vi "get_linearised.vi"(8 "error in (no error)":errorcluster, 11 "ImageCollection in":refnum<class "ImageCollection.lvclass">) -> (0 "error out":errorcluster, 2 "pixels":dbl[](array[numeric]), 3 "ImageCollection out":refnum<class "ImageCollection.lvclass">)   [LabVIEW 2010, in "ImageCollection.lvclass"]
uses:
  ImageCollection.lvclass
  Image/Image/Image.lvclass
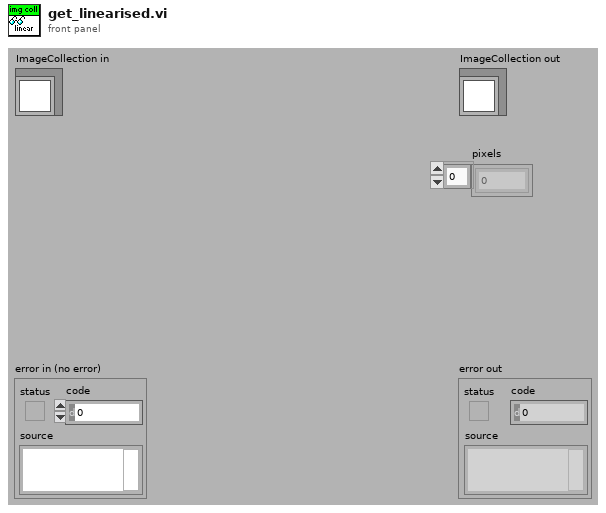
[diagram p1: front panel]
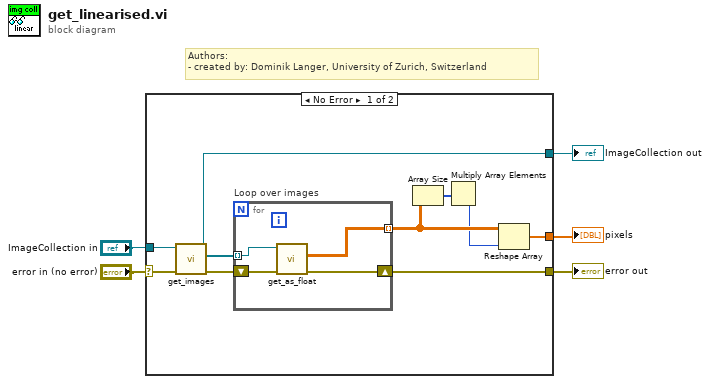
[diagram p0: block diagram]
diagram:
  # "Authors: \n- created by: Dominik Langer, University of Zurich, Switzerland"
  n1 = case shown="No Error" "error in (no error)" {
    selector: "error in (no error)" -> [w15 w21]
    tunnel: [w11 w21] -> w4
    tunnel: [w13 w20] -> w2
    tunnel: "ImageCollection in" -> [w14 w20]
    tunnel: [w9 _] -> w1
    frame No Error {
      n2 = call-dynamic "get_images.vi"("error in (no error)"=w15, "ImageCollection.lvclass in"=w14) -> ("error out"=w12:errorcluster, "images"=w10:refnum<class "Image.lvclass">[], "ImageCollection.lvclass out"=w13:refnum<class "ImageCollection.lvclass">)  [unwired: 7 in]
      n3 = for "Loop over images" {
        shift-right: [w17] -> w11
        shift-left: w12 -> [w19]
        tunnel: w10 -> [w18] mode=indexing
        tunnel: [w16] -> w8 mode=indexing
        n4 = call "get_as_float.vi"("error in (no error)"=w19, "Image in"=w18) -> ("error out"=w17:errorcluster, "data"=w16:sgl[][])  [unwired: 7 in, 1 out]
      }
      n5 = Array Size(array=w8) -> (size(s)=w7:i32[])
      n6 = Multiply Array Elements(1:w7) -> (0:w6:i32)
      n7 = Reshape Array(w8, w6) -> (w9:sgl[])
    }
    frame Error {
    }
  }
  "error out" <- w4
  "ImageCollection out" <- w2
  "pixels" <- w1
